vi "PathPlanner_Holonomic_Execute_Segment.vi"(6 "end time override":dbl, 8 "error in":errorcluster, 11 "inPathPlanner_Holonomic":T1={"HOLONOMIC_DRV_CTRL"={"poseTolerance"={"TRANSLATION"={"X"=0.0, "Y"=0.0}, "ROTATION"={"VALUE"=0.0, "COS"=1.0, "SIN"=0.0}}, "poseError"={"TRANSLATION"={"X"=0.0, "Y"=0.0}, "ROTATION"={"VALUE"=0.0, "COS"=1.0, "SIN"=0.0}}, "Enabled"=TRUE, "PID_xCtrl"={"Kp"=0.0, "Ki"=0.0, "Kd"=0.0, "Period"=0.0, "Max_Integral"=1.0, "Min_Integral"=-1.0, "Max_Input"=0.0, "Min_Input"=0.0, "Continuous"=FALSE, "PositionError"=0.0, "VelocityError"=0.0, "PrevError"=0.0, "TotalError"=0.0, "PositionTolerance"=0.05, "VelocityTolerance"=9.99e+35, "SetPoint"=0.0, "Kf"=0.0, "Prev_Deriv"=0.0, "Prev_Deriv 2"=0.0, "DerivativeFilter"=FALSE, "Min_Output"=-9.99e+35, "Max_Output"=9.9e+35, "Prev_F_P"=0.0, "Prev_F_P_2"=0.0, "AntiWindupActive"=FALSE, "Measurement"=0.0}, "PID_yCtrl"={"Kp"=0.0, "Ki"=0.0, "Kd"=0.0, "Period"=0.0, "Max_Integral"=1.0, "Min_Integral"=-1.0, "Max_Input"=0.0, "Min_Input"=0.0, "Continuous"=FALSE, "PositionError"=0.0, "VelocityError"=0.0, "PrevError"=0.0, "TotalError"=0.0, "PositionTolerance"=0.05, "VelocityTolerance"=9.99e+35, "SetPoint"=0.0, "Kf"=0.0, "Prev_Deriv"=0.0, "Prev_Deriv 2"=0.0, "DerivativeFilter"=FALSE, "Min_Output"=-9.99e+35, "Max_Output"=9.9e+35, "Prev_F_P"=0.0, "Prev_F_P_2"=0.0, "AntiWindupActive"=FALSE, "Measurement"=0.0}, "PROF_PID_thetaCtrl"={"Controller"={"Kp"=0.0, "Ki"=0.0, "Kd"=0.0, "Period"=0.0, "Max_Integral"=1.0, "Min_Integral"=-1.0, "Max_Input"=0.0, "Min_Input"=0.0, "Continuous"=FALSE, "PositionError"=0.0, "VelocityError"=0.0, "PrevError"=0.0, "TotalError"=0.0, "PositionTolerance"=0.05, "VelocityTolerance"=9.99e+35, "SetPoint"=0.0, "Kf"=0.0, "Prev_Deriv"=0.0, "Prev_Deriv 2"=0.0, "DerivativeFilter"=FALSE, "Min_Output"=-9.99e+35, "Max_Output"=9.9e+35, "Prev_F_P"=0.0, "Prev_F_P_2"=0.0, "AntiWindupActive"=FALSE, "Measurement"=0.0}, "Goal"={"Position"=0.0, "Velocity"=0.0}, "Setpoint"={"Position"=0.0, "Velocity"=0.0}, "Constraint"={"MaxVelocity"=0.0, "MaxAcceleration"=0.0}}, "RotationError"={"VALUE"=0.0, "COS"=1.0, "SIN"=0.0}, "FirstRun"=FALSE}, "PathPlannerWayPoints"=[]} {"HOLONOMIC_DRV_CTRL"."RotationError"."SIN" format="%13.4f"; "HOLONOMIC_DRV_CTRL"."RotationError"."COS" format="%13.4f"; "HOLONOMIC_DRV_CTRL"."RotationError"."VALUE" format="%13.4f"; "HOLONOMIC_DRV_CTRL"."PROF_PID_thetaCtrl"."Constraint"."MaxAcceleration" format="%16_6e"; "HOLONOMIC_DRV_CTRL"."PROF_PID_thetaCtrl"."Constraint"."MaxVelocity" format="%16_6e"; "HOLONOMIC_DRV_CTRL"."PROF_PID_thetaCtrl"."Setpoint"."Velocity" format="%16_6e"; "HOLONOMIC_DRV_CTRL"."PROF_PID_thetaCtrl"."Setpoint"."Position" format="%16_6e"; "HOLONOMIC_DRV_CTRL"."PROF_PID_thetaCtrl"."Goal"."Velocity" format="%16_6e"; "HOLONOMIC_DRV_CTRL"."PROF_PID_thetaCtrl"."Goal"."Position" format="%16_6e"; "HOLONOMIC_DRV_CTRL"."PROF_PID_thetaCtrl"."Controller"."Measurement" format="%16_6e"; "HOLONOMIC_DRV_CTRL"."PROF_PID_thetaCtrl"."Controller"."Prev_F_P_2" format="%16_6e"; "HOLONOMIC_DRV_CTRL"."PROF_PID_thetaCtrl"."Controller"."Prev_F_P" format="%16_6e"; "HOLONOMIC_DRV_CTRL"."PROF_PID_thetaCtrl"."Controller"."Max_Output" format="%16_6e"; "HOLONOMIC_DRV_CTRL"."PROF_PID_thetaCtrl"."Controller"."Min_Output" format="%16_6e"; "HOLONOMIC_DRV_CTRL"."PROF_PID_thetaCtrl"."Controller"."Prev_Deriv 2" format="%16_6e"; "HOLONOMIC_DRV_CTRL"."PROF_PID_thetaCtrl"."Controller"."Prev_Deriv" format="%16_6e"; "HOLONOMIC_DRV_CTRL"."PROF_PID_thetaCtrl"."Controller"."Kf" format="%16_6e"; "HOLONOMIC_DRV_CTRL"."PROF_PID_thetaCtrl"."Controller"."SetPoint" format="%16_6e"; "HOLONOMIC_DRV_CTRL"."PROF_PID_thetaCtrl"."Controller"."VelocityTolerance" format="%16_6e"; "HOLONOMIC_DRV_CTRL"."PROF_PID_thetaCtrl"."Controller"."PositionTolerance" format="%16_6e"; "HOLONOMIC_DRV_CTRL"."PROF_PID_thetaCtrl"."Controller"."TotalError" format="%16_6e"; "HOLONOMIC_DRV_CTRL"."PROF_PID_thetaCtrl"."Controller"."PrevError" format="%16_6e"; "HOLONOMIC_DRV_CTRL"."PROF_PID_thetaCtrl"."Controller"."VelocityError" format="%16_6e"; "HOLONOMIC_DRV_CTRL"."PROF_PID_thetaCtrl"."Controller"."PositionError" format="%16_6e"; "HOLONOMIC_DRV_CTRL"."PROF_PID_thetaCtrl"."Controller"."Min_Input" format="%16_6e"; "HOLONOMIC_DRV_CTRL"."PROF_PID_thetaCtrl"."Controller"."Max_Input" format="%16_6e"; "HOLONOMIC_DRV_CTRL"."PROF_PID_thetaCtrl"."Controller"."Min_Integral" format="%16_6e"; "HOLONOMIC_DRV_CTRL"."PROF_PID_thetaCtrl"."Controller"."Max_Integral" format="%16_6e"; "HOLONOMIC_DRV_CTRL"."PROF_PID_thetaCtrl"."Controller"."Period" format="%16_6e"; "HOLONOMIC_DRV_CTRL"."PROF_PID_thetaCtrl"."Controller"."Kd" format="%16_6e"; "HOLONOMIC_DRV_CTRL"."PROF_PID_thetaCtrl"."Controller"."Ki" format="%16_6e"; "HOLONOMIC_DRV_CTRL"."PROF_PID_thetaCtrl"."Controller"."Kp" format="%16_6e"; "HOLONOMIC_DRV_CTRL"."PID_yCtrl"."Measurement" format="%16_6e"; "HOLONOMIC_DRV_CTRL"."PID_yCtrl"."Prev_F_P_2" format="%16_6e"; "HOLONOMIC_DRV_CTRL"."PID_yCtrl"."Prev_F_P" format="%16_6e"; "HOLONOMIC_DRV_CTRL"."PID_yCtrl"."Max_Output" format="%16_6e"; "HOLONOMIC_DRV_CTRL"."PID_yCtrl"."Min_Output" format="%16_6e"; "HOLONOMIC_DRV_CTRL"."PID_yCtrl"."Prev_Deriv 2" format="%16_6e"; "HOLONOMIC_DRV_CTRL"."PID_yCtrl"."Prev_Deriv" format="%16_6e"; "HOLONOMIC_DRV_CTRL"."PID_yCtrl"."Kf" format="%16_6e"; "HOLONOMIC_DRV_CTRL"."PID_yCtrl"."SetPoint" format="%16_6e"; "HOLONOMIC_DRV_CTRL"."PID_yCtrl"."VelocityTolerance" format="%16_6e"; "HOLONOMIC_DRV_CTRL"."PID_yCtrl"."PositionTolerance" format="%16_6e"; "HOLONOMIC_DRV_CTRL"."PID_yCtrl"."TotalError" format="%16_6e"; "HOLONOMIC_DRV_CTRL"."PID_yCtrl"."PrevError" format="%16_6e"; "HOLONOMIC_DRV_CTRL"."PID_yCtrl"."VelocityError" format="%16_6e"; "HOLONOMIC_DRV_CTRL"."PID_yCtrl"."PositionError" format="%16_6e"; "HOLONOMIC_DRV_CTRL"."PID_yCtrl"."Min_Input" format="%16_6e"; "HOLONOMIC_DRV_CTRL"."PID_yCtrl"."Max_Input" format="%16_6e"; "HOLONOMIC_DRV_CTRL"."PID_yCtrl"."Min_Integral" format="%16_6e"; "HOLONOMIC_DRV_CTRL"."PID_yCtrl"."Max_Integral" format="%16_6e"; "HOLONOMIC_DRV_CTRL"."PID_yCtrl"."Period" format="%16_6e"; "HOLONOMIC_DRV_CTRL"."PID_yCtrl"."Kd" format="%16_6e"; "HOLONOMIC_DRV_CTRL"."PID_yCtrl"."Ki" format="%16_6e"; "HOLONOMIC_DRV_CTRL"."PID_yCtrl"."Kp" format="%16_6e"; "HOLONOMIC_DRV_CTRL"."PID_xCtrl"."Measurement" format="%16_6e"; "HOLONOMIC_DRV_CTRL"."PID_xCtrl"."Prev_F_P_2" format="%16_6e"; "HOLONOMIC_DRV_CTRL"."PID_xCtrl"."Prev_F_P" format="%16_6e"; "HOLONOMIC_DRV_CTRL"."PID_xCtrl"."Max_Output" format="%16_6e"; "HOLONOMIC_DRV_CTRL"."PID_xCtrl"."Min_Output" format="%16_6e"; "HOLONOMIC_DRV_CTRL"."PID_xCtrl"."Prev_Deriv 2" format="%16_6e"; "HOLONOMIC_DRV_CTRL"."PID_xCtrl"."Prev_Deriv" format="%16_6e"; "HOLONOMIC_DRV_CTRL"."PID_xCtrl"."Kf" format="%16_6e"; "HOLONOMIC_DRV_CTRL"."PID_xCtrl"."SetPoint" format="%16_6e"; "HOLONOMIC_DRV_CTRL"."PID_xCtrl"."VelocityTolerance" format="%16_6e"; "HOLONOMIC_DRV_CTRL"."PID_xCtrl"."PositionTolerance" format="%16_6e"; "HOLONOMIC_DRV_CTRL"."PID_xCtrl"."TotalError" format="%16_6e"; "HOLONOMIC_DRV_CTRL"."PID_xCtrl"."PrevError" format="%16_6e"; "HOLONOMIC_DRV_CTRL"."PID_xCtrl"."VelocityError" format="%16_6e"; "HOLONOMIC_DRV_CTRL"."PID_xCtrl"."PositionError" format="%16_6e"; "HOLONOMIC_DRV_CTRL"."PID_xCtrl"."Min_Input" format="%16_6e"; "HOLONOMIC_DRV_CTRL"."PID_xCtrl"."Max_Input" format="%16_6e"; "HOLONOMIC_DRV_CTRL"."PID_xCtrl"."Min_Integral" format="%16_6e"; "HOLONOMIC_DRV_CTRL"."PID_xCtrl"."Max_Integral" format="%16_6e"; "HOLONOMIC_DRV_CTRL"."PID_xCtrl"."Period" format="%16_6e"; "HOLONOMIC_DRV_CTRL"."PID_xCtrl"."Kd" format="%16_6e"; "HOLONOMIC_DRV_CTRL"."PID_xCtrl"."Ki" format="%16_6e"; "HOLONOMIC_DRV_CTRL"."PID_xCtrl"."Kp" format="%16_6e"; "HOLONOMIC_DRV_CTRL"."poseError"."ROTATION"."SIN" format="%13.4f"; "HOLONOMIC_DRV_CTRL"."poseError"."ROTATION"."COS" format="%13.4f"; "HOLONOMIC_DRV_CTRL"."poseError"."ROTATION"."VALUE" format="%13.4f"; "HOLONOMIC_DRV_CTRL"."poseError"."TRANSLATION"."Y" format="%14.3f"; "HOLONOMIC_DRV_CTRL"."poseError"."TRANSLATION"."X" format="%14.3f"; "HOLONOMIC_DRV_CTRL"."poseTolerance"."ROTATION"."SIN" format="%13.4f"; "HOLONOMIC_DRV_CTRL"."poseTolerance"."ROTATION"."COS" format="%13.4f"; "HOLONOMIC_DRV_CTRL"."poseTolerance"."ROTATION"."VALUE" format="%13.4f"; "HOLONOMIC_DRV_CTRL"."poseTolerance"."TRANSLATION"."Y" format="%14.3f"; "HOLONOMIC_DRV_CTRL"."poseTolerance"."TRANSLATION"."X" format="%14.3f"; "PathPlannerWayPoints"."HolonomicRotation"."SIN" format="%13.4f"; "PathPlannerWayPoints"."HolonomicRotation"."COS" format="%13.4f"; "PathPlannerWayPoints"."HolonomicRotation"."VALUE" format="%13.4f"; "PathPlannerWayPoints"."NextControl"."Y" format="%14.3f"; "PathPlannerWayPoints"."NextControl"."X" format="%14.3f"; "PathPlannerWayPoints"."PrevControl"."Y" format="%14.3f"; "PathPlannerWayPoints"."PrevControl"."X" format="%14.3f"; "PathPlannerWayPoints"."AnchorPoint"."Y" format="%14.3f"; "PathPlannerWayPoints"."AnchorPoint"."X" format="%14.3f"}) -> (0 "error out":errorcluster, 3 "outPathPlanner_Holonomic":T1={"HOLONOMIC_DRV_CTRL"={"poseTolerance"={"TRANSLATION"={"X"=0.0, "Y"=0.0}, "ROTATION"={"VALUE"=0.0, "COS"=1.0, "SIN"=0.0}}, "poseError"={"TRANSLATION"={"X"=0.0, "Y"=0.0}, "ROTATION"={"VALUE"=0.0, "COS"=1.0, "SIN"=0.0}}, "Enabled"=TRUE, "PID_xCtrl"={"Kp"=0.0, "Ki"=0.0, "Kd"=0.0, "Period"=0.0, "Max_Integral"=1.0, "Min_Integral"=-1.0, "Max_Input"=0.0, "Min_Input"=0.0, "Continuous"=FALSE, "PositionError"=0.0, "VelocityError"=0.0, "PrevError"=0.0, "TotalError"=0.0, "PositionTolerance"=0.05, "VelocityTolerance"=9.99e+35, "SetPoint"=0.0, "Kf"=0.0, "Prev_Deriv"=0.0, "Prev_Deriv 2"=0.0, "DerivativeFilter"=FALSE, "Min_Output"=-9.99e+35, "Max_Output"=9.9e+35, "Prev_F_P"=0.0, "Prev_F_P_2"=0.0, "AntiWindupActive"=FALSE, "Measurement"=0.0}, "PID_yCtrl"={"Kp"=0.0, "Ki"=0.0, "Kd"=0.0, "Period"=0.0, "Max_Integral"=1.0, "Min_Integral"=-1.0, "Max_Input"=0.0, "Min_Input"=0.0, "Continuous"=FALSE, "PositionError"=0.0, "VelocityError"=0.0, "PrevError"=0.0, "TotalError"=0.0, "PositionTolerance"=0.05, "VelocityTolerance"=9.99e+35, "SetPoint"=0.0, "Kf"=0.0, "Prev_Deriv"=0.0, "Prev_Deriv 2"=0.0, "DerivativeFilter"=FALSE, "Min_Output"=-9.99e+35, "Max_Output"=9.9e+35, "Prev_F_P"=0.0, "Prev_F_P_2"=0.0, "AntiWindupActive"=FALSE, "Measurement"=0.0}, "PROF_PID_thetaCtrl"={"Controller"={"Kp"=0.0, "Ki"=0.0, "Kd"=0.0, "Period"=0.0, "Max_Integral"=1.0, "Min_Integral"=-1.0, "Max_Input"=0.0, "Min_Input"=0.0, "Continuous"=FALSE, "PositionError"=0.0, "VelocityError"=0.0, "PrevError"=0.0, "TotalError"=0.0, "PositionTolerance"=0.05, "VelocityTolerance"=9.99e+35, "SetPoint"=0.0, "Kf"=0.0, "Prev_Deriv"=0.0, "Prev_Deriv 2"=0.0, "DerivativeFilter"=FALSE, "Min_Output"=-9.99e+35, "Max_Output"=9.9e+35, "Prev_F_P"=0.0, "Prev_F_P_2"=0.0, "AntiWindupActive"=FALSE, "Measurement"=0.0}, "Goal"={"Position"=0.0, "Velocity"=0.0}, "Setpoint"={"Position"=0.0, "Velocity"=0.0}, "Constraint"={"MaxVelocity"=0.0, "MaxAcceleration"=0.0}}, "RotationError"={"VALUE"=0.0, "COS"=1.0, "SIN"=0.0}, "FirstRun"=FALSE}, "PathPlannerWayPoints"=[]} {"HOLONOMIC_DRV_CTRL"."RotationError"."SIN" format="%13.4f"; "HOLONOMIC_DRV_CTRL"."RotationError"."COS" format="%13.4f"; "HOLONOMIC_DRV_CTRL"."RotationError"."VALUE" format="%13.4f"; "HOLONOMIC_DRV_CTRL"."PROF_PID_thetaCtrl"."Constraint"."MaxAcceleration" format="%16_6e"; "HOLONOMIC_DRV_CTRL"."PROF_PID_thetaCtrl"."Constraint"."MaxVelocity" format="%16_6e"; "HOLONOMIC_DRV_CTRL"."PROF_PID_thetaCtrl"."Setpoint"."Velocity" format="%16_6e"; "HOLONOMIC_DRV_CTRL"."PROF_PID_thetaCtrl"."Setpoint"."Position" format="%16_6e"; "HOLONOMIC_DRV_CTRL"."PROF_PID_thetaCtrl"."Goal"."Velocity" format="%16_6e"; "HOLONOMIC_DRV_CTRL"."PROF_PID_thetaCtrl"."Goal"."Position" format="%16_6e"; "HOLONOMIC_DRV_CTRL"."PROF_PID_thetaCtrl"."Controller"."Measurement" format="%16_6e"; "HOLONOMIC_DRV_CTRL"."PROF_PID_thetaCtrl"."Controller"."Prev_F_P_2" format="%16_6e"; "HOLONOMIC_DRV_CTRL"."PROF_PID_thetaCtrl"."Controller"."Prev_F_P" format="%16_6e"; "HOLONOMIC_DRV_CTRL"."PROF_PID_thetaCtrl"."Controller"."Max_Output" format="%16_6e"; "HOLONOMIC_DRV_CTRL"."PROF_PID_thetaCtrl"."Controller"."Min_Output" format="%16_6e"; "HOLONOMIC_DRV_CTRL"."PROF_PID_thetaCtrl"."Controller"."Prev_Deriv 2" format="%16_6e"; "HOLONOMIC_DRV_CTRL"."PROF_PID_thetaCtrl"."Controller"."Prev_Deriv" format="%16_6e"; "HOLONOMIC_DRV_CTRL"."PROF_PID_thetaCtrl"."Controller"."Kf" format="%16_6e"; "HOLONOMIC_DRV_CTRL"."PROF_PID_thetaCtrl"."Controller"."SetPoint" format="%16_6e"; "HOLONOMIC_DRV_CTRL"."PROF_PID_thetaCtrl"."Controller"."VelocityTolerance" format="%16_6e"; "HOLONOMIC_DRV_CTRL"."PROF_PID_thetaCtrl"."Controller"."PositionTolerance" format="%16_6e"; "HOLONOMIC_DRV_CTRL"."PROF_PID_thetaCtrl"."Controller"."TotalError" format="%16_6e"; "HOLONOMIC_DRV_CTRL"."PROF_PID_thetaCtrl"."Controller"."PrevError" format="%16_6e"; "HOLONOMIC_DRV_CTRL"."PROF_PID_thetaCtrl"."Controller"."VelocityError" format="%16_6e"; "HOLONOMIC_DRV_CTRL"."PROF_PID_thetaCtrl"."Controller"."PositionError" format="%16_6e"; "HOLONOMIC_DRV_CTRL"."PROF_PID_thetaCtrl"."Controller"."Min_Input" format="%16_6e"; "HOLONOMIC_DRV_CTRL"."PROF_PID_thetaCtrl"."Controller"."Max_Input" format="%16_6e"; "HOLONOMIC_DRV_CTRL"."PROF_PID_thetaCtrl"."Controller"."Min_Integral" format="%16_6e"; "HOLONOMIC_DRV_CTRL"."PROF_PID_thetaCtrl"."Controller"."Max_Integral" format="%16_6e"; "HOLONOMIC_DRV_CTRL"."PROF_PID_thetaCtrl"."Controller"."Period" format="%16_6e"; "HOLONOMIC_DRV_CTRL"."PROF_PID_thetaCtrl"."Controller"."Kd" format="%16_6e"; "HOLONOMIC_DRV_CTRL"."PROF_PID_thetaCtrl"."Controller"."Ki" format="%16_6e"; "HOLONOMIC_DRV_CTRL"."PROF_PID_thetaCtrl"."Controller"."Kp" format="%16_6e"; "HOLONOMIC_DRV_CTRL"."PID_yCtrl"."Measurement" format="%16_6e"; "HOLONOMIC_DRV_CTRL"."PID_yCtrl"."Prev_F_P_2" format="%16_6e"; "HOLONOMIC_DRV_CTRL"."PID_yCtrl"."Prev_F_P" format="%16_6e"; "HOLONOMIC_DRV_CTRL"."PID_yCtrl"."Max_Output" format="%16_6e"; "HOLONOMIC_DRV_CTRL"."PID_yCtrl"."Min_Output" format="%16_6e"; "HOLONOMIC_DRV_CTRL"."PID_yCtrl"."Prev_Deriv 2" format="%16_6e"; "HOLONOMIC_DRV_CTRL"."PID_yCtrl"."Prev_Deriv" format="%16_6e"; "HOLONOMIC_DRV_CTRL"."PID_yCtrl"."Kf" format="%16_6e"; "HOLONOMIC_DRV_CTRL"."PID_yCtrl"."SetPoint" format="%16_6e"; "HOLONOMIC_DRV_CTRL"."PID_yCtrl"."VelocityTolerance" format="%16_6e"; "HOLONOMIC_DRV_CTRL"."PID_yCtrl"."PositionTolerance" format="%16_6e"; "HOLONOMIC_DRV_CTRL"."PID_yCtrl"."TotalError" format="%16_6e"; "HOLONOMIC_DRV_CTRL"."PID_yCtrl"."PrevError" format="%16_6e"; "HOLONOMIC_DRV_CTRL"."PID_yCtrl"."VelocityError" format="%16_6e"; "HOLONOMIC_DRV_CTRL"."PID_yCtrl"."PositionError" format="%16_6e"; "HOLONOMIC_DRV_CTRL"."PID_yCtrl"."Min_Input" format="%16_6e"; "HOLONOMIC_DRV_CTRL"."PID_yCtrl"."Max_Input" format="%16_6e"; "HOLONOMIC_DRV_CTRL"."PID_yCtrl"."Min_Integral" format="%16_6e"; "HOLONOMIC_DRV_CTRL"."PID_yCtrl"."Max_Integral" format="%16_6e"; "HOLONOMIC_DRV_CTRL"."PID_yCtrl"."Period" format="%16_6e"; "HOLONOMIC_DRV_CTRL"."PID_yCtrl"."Kd" format="%16_6e"; "HOLONOMIC_DRV_CTRL"."PID_yCtrl"."Ki" format="%16_6e"; "HOLONOMIC_DRV_CTRL"."PID_yCtrl"."Kp" format="%16_6e"; "HOLONOMIC_DRV_CTRL"."PID_xCtrl"."Measurement" format="%16_6e"; "HOLONOMIC_DRV_CTRL"."PID_xCtrl"."Prev_F_P_2" format="%16_6e"; "HOLONOMIC_DRV_CTRL"."PID_xCtrl"."Prev_F_P" format="%16_6e"; "HOLONOMIC_DRV_CTRL"."PID_xCtrl"."Max_Output" format="%16_6e"; "HOLONOMIC_DRV_CTRL"."PID_xCtrl"."Min_Output" format="%16_6e"; "HOLONOMIC_DRV_CTRL"."PID_xCtrl"."Prev_Deriv 2" format="%16_6e"; "HOLONOMIC_DRV_CTRL"."PID_xCtrl"."Prev_Deriv" format="%16_6e"; "HOLONOMIC_DRV_CTRL"."PID_xCtrl"."Kf" format="%16_6e"; "HOLONOMIC_DRV_CTRL"."PID_xCtrl"."SetPoint" format="%16_6e"; "HOLONOMIC_DRV_CTRL"."PID_xCtrl"."VelocityTolerance" format="%16_6e"; "HOLONOMIC_DRV_CTRL"."PID_xCtrl"."PositionTolerance" format="%16_6e"; "HOLONOMIC_DRV_CTRL"."PID_xCtrl"."TotalError" format="%16_6e"; "HOLONOMIC_DRV_CTRL"."PID_xCtrl"."PrevError" format="%16_6e"; "HOLONOMIC_DRV_CTRL"."PID_xCtrl"."VelocityError" format="%16_6e"; "HOLONOMIC_DRV_CTRL"."PID_xCtrl"."PositionError" format="%16_6e"; "HOLONOMIC_DRV_CTRL"."PID_xCtrl"."Min_Input" format="%16_6e"; "HOLONOMIC_DRV_CTRL"."PID_xCtrl"."Max_Input" format="%16_6e"; "HOLONOMIC_DRV_CTRL"."PID_xCtrl"."Min_Integral" format="%16_6e"; "HOLONOMIC_DRV_CTRL"."PID_xCtrl"."Max_Integral" format="%16_6e"; "HOLONOMIC_DRV_CTRL"."PID_xCtrl"."Period" format="%16_6e"; "HOLONOMIC_DRV_CTRL"."PID_xCtrl"."Kd" format="%16_6e"; "HOLONOMIC_DRV_CTRL"."PID_xCtrl"."Ki" format="%16_6e"; "HOLONOMIC_DRV_CTRL"."PID_xCtrl"."Kp" format="%16_6e"; "HOLONOMIC_DRV_CTRL"."poseError"."ROTATION"."SIN" format="%13.4f"; "HOLONOMIC_DRV_CTRL"."poseError"."ROTATION"."COS" format="%13.4f"; "HOLONOMIC_DRV_CTRL"."poseError"."ROTATION"."VALUE" format="%13.4f"; "HOLONOMIC_DRV_CTRL"."poseError"."TRANSLATION"."Y" format="%14.3f"; "HOLONOMIC_DRV_CTRL"."poseError"."TRANSLATION"."X" format="%14.3f"; "HOLONOMIC_DRV_CTRL"."poseTolerance"."ROTATION"."SIN" format="%13.4f"; "HOLONOMIC_DRV_CTRL"."poseTolerance"."ROTATION"."COS" format="%13.4f"; "HOLONOMIC_DRV_CTRL"."poseTolerance"."ROTATION"."VALUE" format="%13.4f"; "HOLONOMIC_DRV_CTRL"."poseTolerance"."TRANSLATION"."Y" format="%14.3f"; "HOLONOMIC_DRV_CTRL"."poseTolerance"."TRANSLATION"."X" format="%14.3f"; "PathPlannerWayPoints"."HolonomicRotation"."SIN" format="%13.4f"; "PathPlannerWayPoints"."HolonomicRotation"."COS" format="%13.4f"; "PathPlannerWayPoints"."HolonomicRotation"."VALUE" format="%13.4f"; "PathPlannerWayPoints"."NextControl"."Y" format="%14.3f"; "PathPlannerWayPoints"."NextControl"."X" format="%14.3f"; "PathPlannerWayPoints"."PrevControl"."Y" format="%14.3f"; "PathPlannerWayPoints"."PrevControl"."X" format="%14.3f"; "PathPlannerWayPoints"."AnchorPoint"."Y" format="%14.3f"; "PathPlannerWayPoints"."AnchorPoint"."X" format="%14.3f"})   [LabVIEW 2020]
doc: "Executes the next segment of a <B>PathPlanner</B> trajectory."
uses:
  PathPlanner_Holonomic.ctl
  <vilib>/Rock Robotics/WPI/ThirdParty/JAS_Junk/TrajLib/HOLONOMIC_DRV_CTRL.ctl
  <vilib>/Rock Robotics/WPI/ThirdParty/JAS_Junk/TrajLib/POSE2D.ctl
  <vilib>/Rock Robotics/WPI/ThirdParty/JAS_Junk/TrajLib/TRANSLATION2D.ctl
  <vilib>/Rock Robotics/WPI/ThirdParty/JAS_Junk/TrajLib/ROTATION2D.ctl
  <vilib>/Rock Robotics/WPI/ThirdParty/JAS_Junk/TrajLib/PID_CONTROLLER.ctl
  <vilib>/Rock Robotics/WPI/ThirdParty/JAS_Junk/TrajLib/PROFILED_PID_CONTROLLER.ctl
  <vilib>/Rock Robotics/WPI/ThirdParty/JAS_Junk/TrajLib/TRAPEZOID_PROFILE_STATE.ctl
  <vilib>/Rock Robotics/WPI/ThirdParty/JAS_Junk/TrajLib/TRAPEZOID_PROFILE_CONSTRAINT.ctl
  <vilib>/Rock Robotics/WPI/ThirdParty/MJansen/PathPlanner/PathPlannerWaypoint.ctl
  HolDrvCtrl_Calculate_FIXED.vi
  <vilib>/Rock Robotics/WPI/ThirdParty/JAS_Junk/TrajLib/ProfiledPIDController_Calculate_Meas_Goal.vi
  <vilib>/Rock Robotics/WPI/ThirdParty/JAS_Junk/TrajLib/ChassisSpeeds_FromFieldRelativeSpeeds.vi
  <vilib>/Rock Robotics/WPI/ThirdParty/JAS_Junk/TrajLib/PIDController_Reset.vi
  <vilib>/Rock Robotics/WPI/ThirdParty/JAS_Junk/TrajLib/PIDController_Calculate_SP_PV.vi
  <vilib>/Rock Robotics/WPI/ThirdParty/JAS_Junk/TrajLib/ProfiledPIDController_Reset_PosOnly.vi
  <vilib>/Rock Robotics/WPI/ThirdParty/JAS_Junk/TrajLib/Pose_getXYAngle.vi
  <vilib>/Rock Robotics/WPI/ThirdParty/JAS_Junk/TrajLib/Rotation_GetAngleCosSin.vi
  <vilib>/Rock Robotics/WPI/ThirdParty/JAS_Junk/TrajLib/Pose_RelativeTo.vi
  <vilib>/Rock Robotics/WPI/ThirdParty/JAS_Junk/TrajLib/Pose_getRotation.vi
  <vilib>/Rock Robotics/WPI/ThirdParty/JAS_Junk/TrajLib/Rotation_Minus.vi
  <vilib>/Rock Robotics/WPI/ThirdParty/JAS_Junk/TrajLib/ProfiledPIDController_SetGoal_PosOnly.vi
  <vilib>/Rock Robotics/WPI/ThirdParty/JAS_Junk/TrajLib/ProfiledPIDController_Calculate_Meas.vi
  <vilib>/Rock Robotics/WPI/ThirdParty/JAS_Junk/TrajLib/Rotation_GetCos.vi
  <vilib>/Rock Robotics/WPI/ThirdParty/JAS_Junk/TrajLib/Rotation_GetSin.vi
  <vilib>/Rock Robotics/WPI/ThirdParty/JAS_Junk/TrajLib/ChassisSpeeds_New.vi
  <vilib>/Rock Robotics/WPI/ThirdParty/JAS_Junk/TrajLib/PIDController_SetSetpoint.vi
  <vilib>/Rock Robotics/WPI/ThirdParty/JAS_Junk/TrajLib/PIDController_Calculate_PV.vi
  <vilib>/Rock Robotics/WPI/ThirdParty/JAS_Junk/TrajLib/TrapProfState_New.vi
  <vilib>/Rock Robotics/WPI/ThirdParty/JAS_Junk/TrajLib/ProfiledPIDController_Reset.vi
  <vilib>/Rock Robotics/WPI/ThirdParty/JAS_Junk/TrajLib/Transform_Create_PosePose.vi
  <vilib>/Rock Robotics/WPI/ThirdParty/JAS_Junk/TrajLib/Pose_New_TRRO.vi
  <vilib>/Rock Robotics/WPI/ThirdParty/JAS_Junk/TrajLib/Rotation_UnaryMinus.vi
  <vilib>/Rock Robotics/WPI/ThirdParty/JAS_Junk/TrajLib/Rotation_RotateBy.vi
  <vilib>/Rock Robotics/WPI/ThirdParty/JAS_Junk/TrajLib/ProfiledPIDController_SetGoal.vi
  <vilib>/Rock Robotics/WPI/ThirdParty/JAS_Junk/TrajLib/TrapProfile_New.vi
  <vilib>/Rock Robotics/WPI/ThirdParty/JAS_Junk/TrajLib/ProfiledPIDController_GetPeriod.vi
  <vilib>/Rock Robotics/WPI/ThirdParty/JAS_Junk/TrajLib/TrapProfile_Calculate.vi
  <vilib>/Rock Robotics/WPI/ThirdParty/JAS_Junk/TrajLib/ControllerUtil_GetModulusError.vi
  <vilib>/Rock Robotics/WPI/ThirdParty/JAS_Junk/TrajLib/Translation_RotateBy.vi
  <vilib>/Rock Robotics/WPI/ThirdParty/JAS_Junk/TrajLib/Translation_Minus.vi
  <vilib>/Rock Robotics/WPI/ThirdParty/JAS_Junk/TrajLib/Rotation_CreateAngle.vi
  <vilib>/Rock Robotics/WPI/ThirdParty/JAS_Junk/TrajLib/Rotation_CreateXY.vi
  <vilib>/Rock Robotics/WPI/ThirdParty/JAS_Junk/TrajLib/TrapProfile_ShouldFlipAcceleration.vi
  <vilib>/Rock Robotics/WPI/ThirdParty/JAS_Junk/TrajLib/TrapProfile_Direct.vi
  <vilib>/Rock Robotics/SystemInterfaces/NetworkCommunication/NetComm_UsageReport_report.vi
  <vilib>/Rock Robotics/WPI/ThirdParty/JAS_Junk/TrajLib/PIDController_GetPeriod.vi
  <vilib>/Rock Robotics/WPI/ThirdParty/JAS_Junk/TrajLib/Translation_Create.vi
  <vilib>/Rock Robotics/WPI/ThirdParty/JAS_Junk/TrajLib/Util_CalcDist.vi
  <vilib>/Utility/error.llb/Error Cluster From Error Code.vi
  <vilib>/Utility/semaphor.llb/Obtain Semaphore Reference.vi
  <vilib>/Rock Robotics/WPI/ThirdParty/JAS_Junk/TrajLib/Timer_Reset.vi
  Robot Global Data.vi
  Subsystems/Swerve/swerve_globals.vi
  <vilib>/Rock Robotics/WPI/ThirdParty/JAS_Junk/TrajLib/Util_LibraryGlobals.vi
  <vilib>/ErrorRing/Error Ring.xnode
  <vilib>/Rock Robotics/WPI/ThirdParty/JAS_Junk/TrajLib/Trajectory_Library.lvlib
  <vilib>/Rock Robotics/WPI/ThirdParty/MJansen/PathPlanner/PathPlanner.lvlib
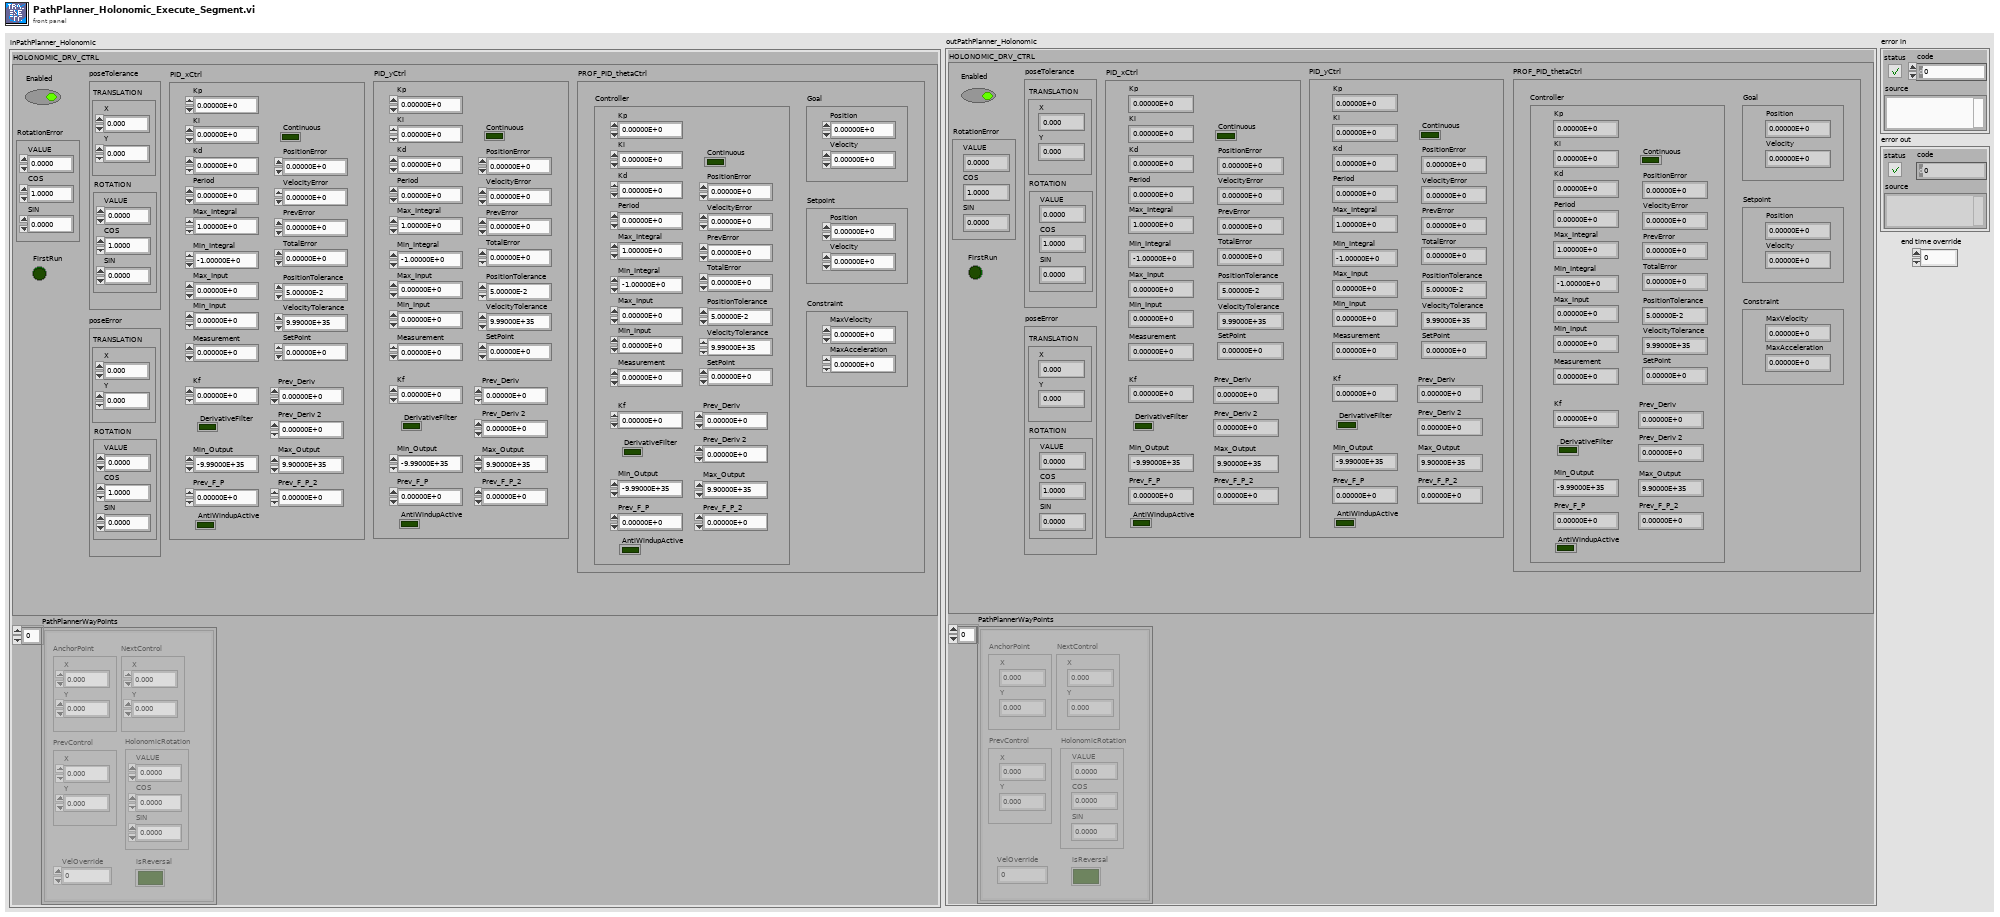
[diagram p1: front panel]
types:
  T1 = typedef "PathPlanner_Holonomic.ctl" = cluster{"HOLONOMIC_DRV_CTRL":T2, "PathPlannerWayPoints":T10[]}
  T2 = typedef "Trajectory_Library.lvlib/HOLONOMIC_DRV_CTRL.ctl" = cluster{"poseTolerance":T3, "poseError":T3, "Enabled":bool, "PID_xCtrl":T6, "PID_yCtrl":T6, "PROF_PID_thetaCtrl":T7, "RotationError":T5, "FirstRun":bool}
  T3 = typedef "Trajectory_Library.lvlib/POSE2D.ctl" = cluster{"TRANSLATION":T4, "ROTATION":T5}
  T4 = typedef "Trajectory_Library.lvlib/TRANSLATION2D.ctl" = cluster{"X":dbl, "Y":dbl}
  T5 = typedef "Trajectory_Library.lvlib/ROTATION2D.ctl" = cluster{"VALUE":dbl, "COS":dbl, "SIN":dbl}
  T6 = typedef "Trajectory_Library.lvlib/PID_CONTROLLER.ctl" = cluster{"Kp":dbl, "Ki":dbl, "Kd":dbl, "Period":dbl, "Max_Integral":dbl, "Min_Integral":dbl, "Max_Input":dbl, "Min_Input":dbl, "Continuous":bool, "PositionError":dbl, "VelocityError":dbl, "PrevError":dbl, "TotalError":dbl, "PositionTolerance":dbl, "VelocityTolerance":dbl, "SetPoint":dbl, "Kf":dbl, "Prev_Deriv":dbl, "Prev_Deriv 2":dbl, "DerivativeFilter":bool, "Min_Output":dbl, "Max_Output":dbl, "Prev_F_P":dbl, "Prev_F_P_2":dbl, "AntiWindupActive":bool, "Measurement":dbl}
  T7 = typedef "Trajectory_Library.lvlib/PROFILED_PID_CONTROLLER.ctl" = cluster{"Controller":T6, "Goal":T8, "Setpoint":T8, "Constraint":T9}
  T8 = typedef "Trajectory_Library.lvlib/TRAPEZOID_PROFILE_STATE.ctl" = cluster{"Position":dbl, "Velocity":dbl}
  T9 = typedef "Trajectory_Library.lvlib/TRAPEZOID_PROFILE_CONSTRAINT.ctl" = cluster{"MaxVelocity":dbl, "MaxAcceleration":dbl}
  T10 = typedef "PathPlanner.lvlib/PathPlannerWaypoint.ctl" = cluster{"AnchorPoint":T4, "PrevControl":T4, "NextControl":T4, "HolonomicRotation":T5, "VelOverride":dbl, "isReversal":bool}
  T11 = typedef "PathPlanner.lvlib/PathPlannerTrajectory.ctl" = cluster{"TotalTimeSeconds":dbl, "States":T12[]}
  T12 = typedef "PathPlanner.lvlib/PathPlannerState.ctl" = cluster{"AngularAcceleration":T5, "PositionMeters":dbl, "TrajectoryState":T13, "AngularVelocity":T5, "HolonomicRotation":T5, "CurveRadius":dbl, "DeltaPos":dbl}
  T13 = typedef "Trajectory_Library.lvlib/TRAJ_STATE.ctl" = cluster{"TimeSeconds":dbl, "Velocity":dbl, "Acceleration":dbl, "POSE":T3, "Curvature":dbl}
  T14 = typedef "Trajectory_Library.lvlib/TIMER.ctl" = cluster{"StartTime":dbl, "Accumulated TIme":dbl, "Running":bool, "semaphore":T15}
  T15 = typedef "Semaphore RefNum" = refnum<k1>
  T16 = typedef "Trajectory_Library.lvlib/CHASSIS_SPEEDS.ctl" = cluster{"vX":dbl, "vY":dbl, "vOmega":dbl}
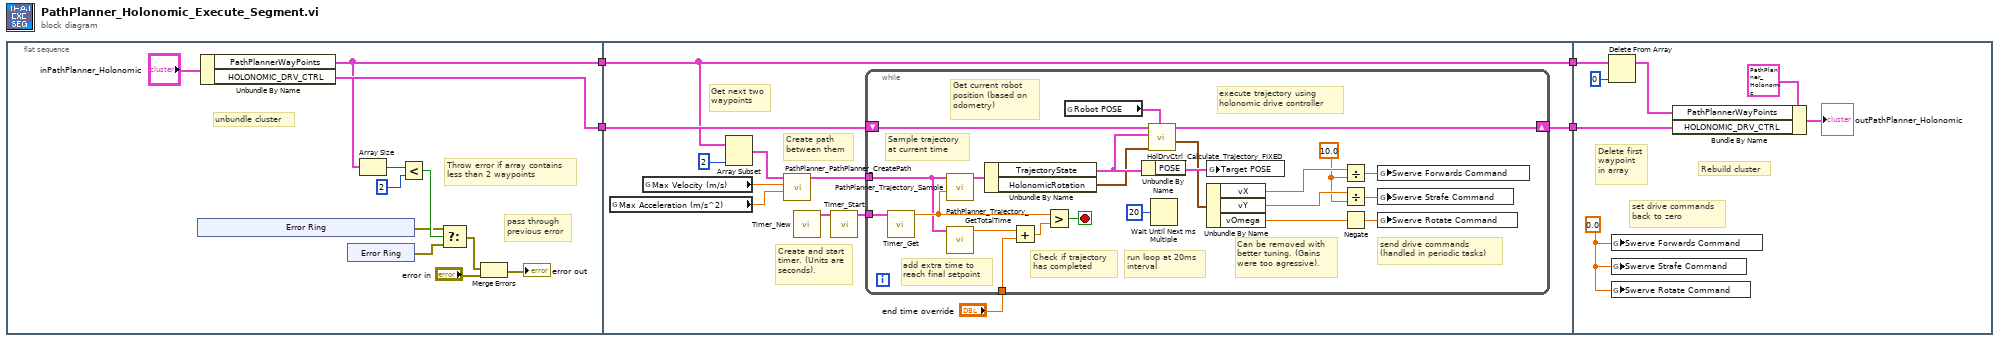
[diagram p0: block diagram]
diagram:
  n1 = flat-sequence {
    tunnel: [w6] -> w3
    tunnel: [w5] -> w1
    tunnel: [w30] -> w4
    tunnel: w3 -> [w31]
    tunnel: [w21] -> w2
    tunnel: w1 -> [w21]
    tunnel: w4 -> [w59]
    tunnel: w2 -> [w57]
    frame #0 {
      # "pass through\nprevious error"
      # "unbundle cluster"
      # "Throw error if array contains\nless than 2 waypoints"
      n2 = xnode "Error Ring"() -> ("error out"=w9:errorcluster)
      n3 = Unbundle By Name("inPathPlanner_Holonomic") -> ("PathPlannerWayPoints"=w5:T10[], "HOLONOMIC_DRV_CTRL"=w6:T2)
      n4 = xnode "Error Ring"() -> ("error out"=w10:errorcluster)
      n5 = Array Size(array=w5) -> (size(s)=w14:i32)
      n6 = Less?(x=w14, y=2) -> (x < y?=w15:bool)
      n7 = Select(t=w9, s=w15, f=w10) -> (s? t:f=w12:errorcluster)
      n8 = Merge Errors(w12, "error in") -> (→"error out":errorcluster)
    }
    frame #1 {
      # "Create and start\ntimer. (Units are\nseconds)."
      # "Create path\nbetween them"
      # "Get next two\nwaypoints"
      n9 = global read "Robot Global Data.vi" "Max Acceleration (m/s^2)"() -> (w25:dbl)
      n10 = global read "Robot Global Data.vi" "Max Velocity (m/s)"() -> (w26:dbl)
      n11 = Array Subset(array=w21, length=2) -> (w28:T10[])  [unwired: 1 in]
      n12 = call <vilib>:"PathPlanner_PathPlanner_CreatePath.vi"("MaxAcceleration"=w25, "MaxVelocity"=w26, "PathPlannerWayPoints"=w28) -> ("PathPlannerTrajectory"=w23:T11)  [unwired: 8 in]
      n13 = call <vilib>:"Timer_New.vi"() -> ("TIMER"=w27:T14)  [unwired: 11 in]
      n14 = call <vilib>:"Timer_Start.vi"("in Timer"=w27) -> ("out Timer"=w22:T14)  [unwired: 10 in]
      n15 = while {
        tunnel: w22 -> [w54]
        shift-right: [w41] -> w30
        shift-left: w31 -> [w51]
        tunnel: w23 -> [w40]
        tunnel: "end time override" -> [w34]
        stop <- w38 stop-if-true
        w42 = 10.0 ("y")
        # "Get current robot\nposition (based on\nodometry)"
        # "add extra time to\nreach final setpoint"
        # "Can be removed with\nbetter tuning. (Gains\nwere too agressive)."
        # "send drive commands\n(handled in periodic tasks)"
        # "execute trajectory using\nholonomic drive controller"
        # "run loop at 20ms\ninterval"
        # "Check if trajectory\nhas completed"
        # "Sample trajectory\nat current time"
        n16 = call <vilib>:"Timer_Get.vi"("TIMER"=w54) -> ("CurrentTImer"=w49:dbl)  [unwired: 10 in]
        n17 = call <vilib>:"PathPlanner_Trajectory_Sample.vi"("Time"=w49, "PathPlannerTrajectory"=w40) -> ("PathPlannerState"=w53:T12)  [unwired: 9 in]
        n18 = call <vilib>:"PathPlanner_Trajectory_GetTotalTime.vi"("PathPlannerTrajectory"=w40) -> ("TotalTimeSeconds"=w39:dbl)  [unwired: 10 in]
        n19 = Unbundle By Name(w53) -> ("TrajectoryState"=w37:T13, "HolonomicRotation"=w36:T5)
        n20 = Add(x=w39, y=w34) -> (x+y=w35:dbl)
        n21 = Greater?(x=w49, y=w35) -> (0:w38:bool)
        n22 = global read "swerve_globals.vi" "Robot POSE"() -> (w52:T3)
        n23 = Unbundle By Name(w37) -> ("POSE"=w48:T3)
        n24 = call "HolDrvCtrl_Calculate_Trajectory_FIXED.vi"("currentPose"=w52, "angleRef"=w36, "desiredTrajState"=w37, "inHOLONOMIC_DRV_CTRL"=w51) -> ("calcChassisSpeed"=w47:T16, "outHOLONOMIC_DRV_CTRL"=w41:T2)  [unwired: 6 in]
        n25 = Wait Until Next ms Multiple(millisecond multiple=u32 20) -> ()  [unwired: 1 out]
        n26 = global write "swerve_globals.vi" "Target POSE"(w48) -> ()
        n27 = Unbundle By Name(w47) -> ("vX"=w46:dbl, "vY"=w45:dbl, "vOmega"=w33:dbl)
        n28 = Divide(x=w46, y=w42) -> (x/y=w43:dbl)
        n29 = Divide(x=w45, y=w42) -> (x/y=w44:dbl)
        n30 = Negate(x=w33) -> (-x=w32:dbl)
        n31 = global write "swerve_globals.vi" "Swerve Forwards Command"(w43) -> ()
        n32 = global write "swerve_globals.vi" "Swerve Strafe Command"(w44) -> ()
        n33 = global write "swerve_globals.vi" "Swerve Rotate Command"(w32) -> ()
      }
    }
    frame #2 {
      w55 = 0.0 ("Swerve Forwards Command")
      # "Rebuild cluster"
      # "set drive commands\nback to zero"
      # "Delete first\nwaypoint\nin array"
      n34 = Delete From Array(array=w57, index=0) -> (array with subset deleted=w56:T10[])  [unwired: 1 in, 1 out]
      n35 = global write "swerve_globals.vi" "Swerve Forwards Command"(w55) -> ()
      n36 = global write "swerve_globals.vi" "Swerve Strafe Command"(w55) -> ()
      n37 = global write "swerve_globals.vi" "Swerve Rotate Command"(w55) -> ()
      n38 = Bundle By Name(cluster=T1 {"HOLONOMIC_DRV_CTRL"={"poseTolerance"={"TRANSLATION"={"X"=0.0, "Y"=0.0}, "ROTATION"={"VALUE"=0.0, "COS"=1.0, "SIN"=0.0}}, "poseError"={"TRANSLATION"={"X"=0.0, "Y"=0.0}, "ROTATION"={"VALUE"=0.0, "COS"=1.0, "SIN"=0.0}}, "Enabled"=TRUE, "PID_xCtrl"={"Kp"=0.0, "Ki"=0.0, "Kd"=0.0, "Period"=0.0, "Max_Integral"=1.0, "Min_Integral"=-1.0, "Max_Input"=0.0, "Min_Input"=0.0, "Continuous"=FALSE, "PositionError"=0.0, "VelocityError"=0.0, "PrevError"=0.0, "TotalError"=0.0, "PositionTolerance"=0.05, "VelocityTolerance"=9.99e+35, "SetPoint"=0.0, "Kf"=0.0, "Prev_Deriv"=0.0, "Prev_Deriv 2"=0.0, "DerivativeFilter"=FALSE, "Min_Output"=-9.99e+35, "Max_Output"=9.9e+35, "Prev_F_P"=0.0, "Prev_F_P_2"=0.0, "AntiWindupActive"=FALSE, "Measurement"=0.0}, "PID_yCtrl"={"Kp"=0.0, "Ki"=0.0, "Kd"=0.0, "Period"=0.0, "Max_Integral"=1.0, "Min_Integral"=-1.0, "Max_Input"=0.0, "Min_Input"=0.0, "Continuous"=FALSE, "PositionError"=0.0, "VelocityError"=0.0, "PrevError"=0.0, "TotalError"=0.0, "PositionTolerance"=0.05, "VelocityTolerance"=9.99e+35, "SetPoint"=0.0, "Kf"=0.0, "Prev_Deriv"=0.0, "Prev_Deriv 2"=0.0, "DerivativeFilter"=FALSE, "Min_Output"=-9.99e+35, "Max_Output"=9.9e+35, "Prev_F_P"=0.0, "Prev_F_P_2"=0.0, "AntiWindupActive"=FALSE, "Measurement"=0.0}, "PROF_PID_thetaCtrl"={"Controller"={"Kp"=0.0, "Ki"=0.0, "Kd"=0.0, "Period"=0.0, "Max_Integral"=1.0, "Min_Integral"=-1.0, "Max_Input"=0.0, "Min_Input"=0.0, "Continuous"=FALSE, "PositionError"=0.0, "VelocityError"=0.0, "PrevError"=0.0, "TotalError"=0.0, "PositionTolerance"=0.05, "VelocityTolerance"=9.99e+35, "SetPoint"=0.0, "Kf"=0.0, "Prev_Deriv"=0.0, "Prev_Deriv 2"=0.0, "DerivativeFilter"=FALSE, "Min_Output"=-9.99e+35, "Max_Output"=9.9e+35, "Prev_F_P"=0.0, "Prev_F_P_2"=0.0, "AntiWindupActive"=FALSE, "Measurement"=0.0}, "Goal"={"Position"=0.0, "Velocity"=0.0}, "Setpoint"={"Position"=0.0, "Velocity"=0.0}, "Constraint"={"MaxVelocity"=0.0, "MaxAcceleration"=0.0}}, "RotationError"={"VALUE"=0.0, "COS"=1.0, "SIN"=0.0}, "FirstRun"=FALSE}, "PathPlannerWayPoints"=[]}, "PathPlannerWayPoints"=w56, "HOLONOMIC_DRV_CTRL"=w59) -> (→"outPathPlanner_Holonomic":T1)
    }
  }
